vi "Send Stop Polling Msg.vi"(8 "error in (no error)":errorcluster, 11 "Message Queue":refnum<queue>) -> (0 "error out":errorcluster, 3 "Message Queue":refnum<queue>)   [LabVIEW 2024, in "Zero Timeout Message Handler.lvlib" / "Stop Polling Msg.lvclass"]
uses:
  Stop Polling Msg.lvclass
  Stop Polling Msg.lvclass/Stop Polling Msg.ctl
  C:/Users/uspoaotto/OneDrive - Oregon Tool/Desktop/working copies/zeroTimeoutMessageHandler/src/Zero Timeout Message Handler/Stop Polling Msg/Stop Polling Msg.lvclass
  C:/Users/uspoaotto/OneDrive - Oregon Tool/Desktop/working copies/zeroTimeoutMessageHandler/src/Zero Timeout Message Handler/~Message/~Message.lvclass
  ~Message/~Message.lvclass
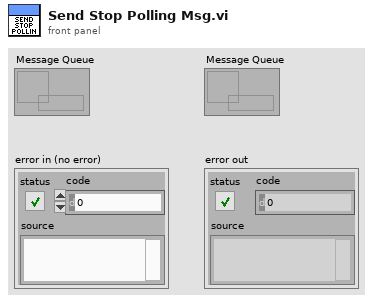
[diagram p1: front panel]
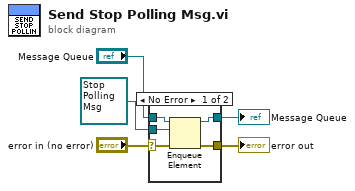
[diagram p0: block diagram]
diagram:
  n1 = case shown="No Error" "error in (no error)" {
    selector: "error in (no error)" -> [w7 w12]
    tunnel: "Message Queue" -> [w10 w11]
    tunnel: [w9 w12] -> w4
    tunnel: refnum<class "Stop Polling Msg.lvclass"> refnum ("Zero Timeout Message Handler.lvlib:Stop Polling Msg.lvclass") -> [w8 _]
    tunnel: [w6 w11] -> w1
    frame No Error {
      n2 = Enqueue Element(queue=w10, element=w8, error in (no error)=w7) -> (queue out=w6:refnum<queue>, error out=w9:errorcluster)  [unwired: 1 in, 1 out]
    }
    frame Error {
    }
  }
  "error out" <- w4
  "Message Queue" <- w1
